vi "Set Copyright.vi"(9 "Company Name":string="Good Automation, LLC", 11 "Current Copyright":string) -> (3 "Updated Copyright":string)   [LabVIEW 2014]
doc: "<b>VI Description:</b> This VI is used to build/update the copyright information of a VI. \n<b>VI Version:</b> 1.0.5.beta \n<b>Review Date:</b> 03/09/2012 \n<b>Author:</b> Jason Willis, Ryan Podsim \n<b>Copyright:</b> Copyright © 2012-2014"
uses:
  <vilib>/regexp/Match Regular Expression.xnode
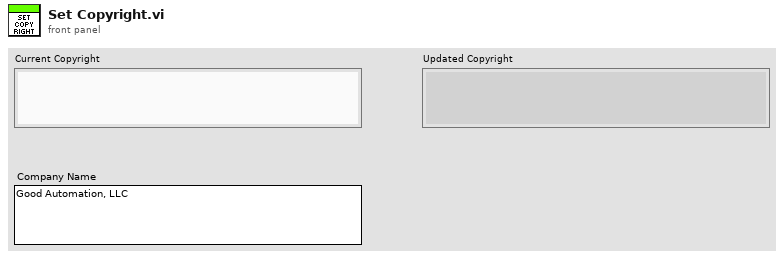
[diagram p1: front panel]
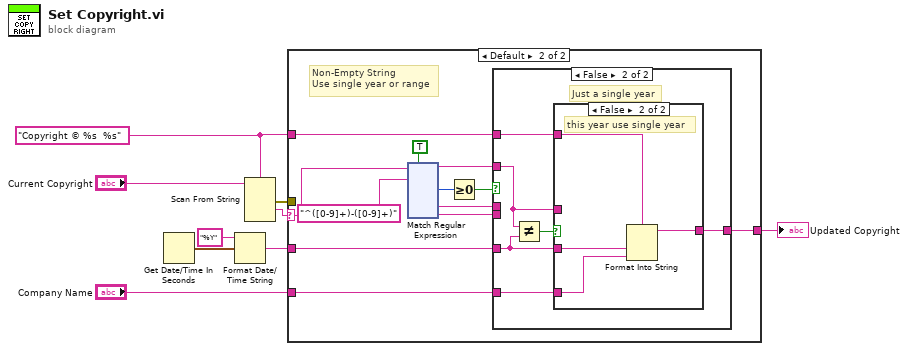
[diagram p0: block diagram]
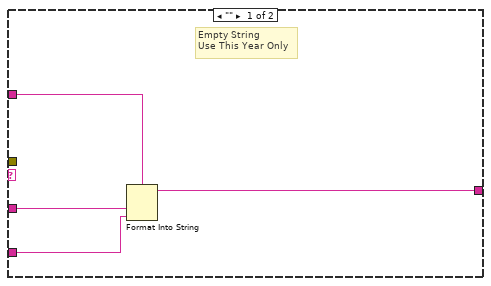
[diagram p2: hidden frame]
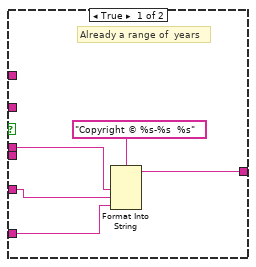
[diagram p3: hidden frame]
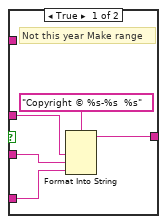
[diagram p4: hidden frame]
diagram:
  w3 = "Copyright © %s  %s"
  n1 = Get Date/Time In Seconds() -> (seconds since 1Jan1904=w8:timestamp)
  n2 = Format Date/Time String(time format string (%c)="%Y", seconds (now)=w8) -> (date/time string=w9:string)  [unwired: 1 in]
  n3 = Scan From String(format string=w3, input string="Current Copyright") -> (error out=w6:errorcluster, output 1=w1:string)  [unwired: 5 in, 2 out]
  n4 = case shown="Default" w1 {
    selector: w1 -> [_ w15]
    tunnel: "Company Name" -> [w13 w24]
    tunnel: [w12 w25] -> w4
    tunnel: w9 -> [w11 w23]
    tunnel: w6 -> [_ _]
    tunnel: w3 -> [w10 w14]
    frame "" {
      # "Empty String\nUse This Year Only"
      n5 = Format Into String(format string=w10, w11, w13) -> (resulting string=w12:string)  [unwired: 2 in, 1 out]
    }
    frame Default {
      # "Non-Empty String\nUse single year or range"
      n6 = xnode "Match Regular Expression"("input string"=w15, "regular expression"="^([0-9]+)-([0-9]+)", "ignore case? (F)"=TRUE) -> ("before match"=w16:string, "offset past match"=w20:i32, "submatch 1"=w19:string, "submatch 2"=w18:string)  [unwired: 3 in, 3 out]
      n7 = Greater Or Equal To 0?(x=w20) -> (x >= 0?=w17:bool)
      n8 = case shown="False" w17 {
        tunnel: [w30 w36] -> w25
        tunnel: w24 -> [w29 w35]
        tunnel: w23 -> [w28 w34]
        tunnel: w16 -> [_ w31]
        tunnel: w19 -> [w27 _]
        tunnel: w18 -> [_ _]
        tunnel: w14 -> [_ w32]
        frame True {
          # "Already a range of  years"
          n9 = Format Into String(format string="Copyright © %s-%s  %s", w27, w28, w29) -> (resulting string=w30:string)  [unwired: 2 in, 1 out]
        }
        frame False {
          # "Just a single year"
          n10 = Not Equal?(x=w31, y=w34) -> (x != y?=w33:bool)
          n11 = case shown="False" w33 {
            tunnel: [w40 w45] -> w36
            tunnel: w35 -> [w39 w44]
            tunnel: w34 -> [w38 w43]
            tunnel: w32 -> [_ w42]
            tunnel: w31 -> [w37 _]
            frame True {
              # "Not this year Make range"
              n12 = Format Into String(format string="Copyright © %s-%s  %s", w37, w38, w39) -> (resulting string=w40:string)  [unwired: 2 in, 1 out]
            }
            frame False {
              # "this year use single year"
              n13 = Format Into String(format string=w42, w43, w44) -> (resulting string=w45:string)  [unwired: 2 in, 1 out]
            }
          }
        }
      }
    }
  }
  "Updated Copyright" <- w4
